vi "Is Mouse in Image Area.vi"(8 "Error In":errorcluster, 10 "Mouse Coords":T2, 11 "Image Control Refnum":T1) -> (0 "Error Out":errorcluster, 3 "Is in Image Area?":bool)   [LabVIEW 2021, in "Image.lvlib"]
uses:
  <vilib>/Utility/miscctls.llb/LVPoint32TypeDef.ctl
  Image Control Refnum.ctl
  Image.lvlib
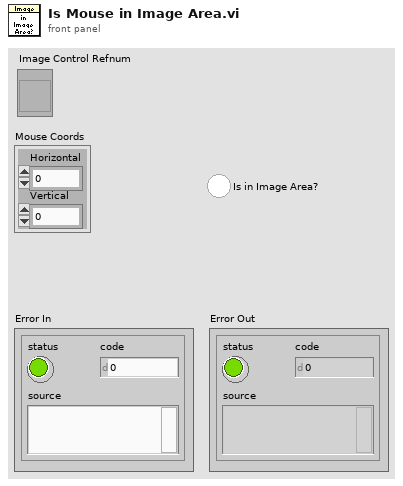
[diagram p1: front panel]
types:
  T1 = typedef "Image.lvlib/Image Control Refnum.ctl" = refnum<vi>
  T2 = typedef "LVPoint32TypeDef.ctl" = cluster{"Horizontal":i32, "Vertical":i32}
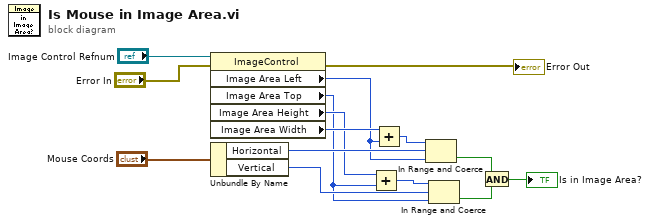
[diagram p0: block diagram]
diagram:
  n1 = property class="ImageControl"(reference="Image Control Refnum", error in="Error In") -> (error out=→"Error Out":errorcluster, "Image Area Left"=w10:i32, "Image Area Top"=w6:i32, "Image Area Height"=w7:u32, "Image Area Width"=w11:u32)  [unwired: 1 out]
  n2 = Unbundle By Name("Mouse Coords") -> ("Horizontal"=w12:i32, "Vertical"=w8:i32)
  n3 = Add(x=w7, y=w6) -> (x+y=w5:u32)
  n4 = Add(x=w11, y=w10) -> (x+y=w9:u32)
  n5 = In Range and Coerce(upper limit=w9, x=w12, lower limit=w10) -> (In Range?=w4:bool)  [unwired: 1 out]
  n6 = In Range and Coerce(upper limit=w5, x=w8, lower limit=w6) -> (In Range?=w3:bool)  [unwired: 1 out]
  n7 = And(x=w4, y=w3) -> (x .and. y?=→"Is in Image Area?":bool)
